vi "TDMS write test.vi"   [LabVIEW 2013]
types:
  T1 = enum16{"open", "open or create", "create or replace", "create", "open (read-only)"}
  T2 = typedef "electrical.ctl" = cluster{"date/time string":string, "Electrical Data Labels":string[], "Electrical Data":string[], "Waveform Graph":waveform(dbl)[]}
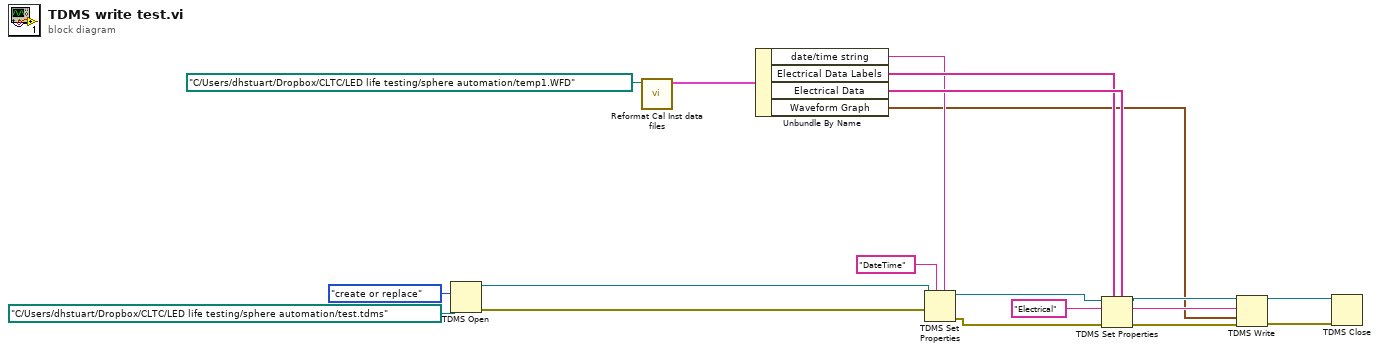
[diagram p0: block diagram]
diagram:
  n1 = TDMS Open(10:T1."create or replace" ("operation (0:open)"), 11:path "C:/Users/dhstuart/Dropbox/CLTC/LED life testing/sphere automation/test.tdms" ("file path")) -> (0:w17:errorcluster, 3:w18:refnum<k34>)  [unwired: 5 in]
  n2 = call "Reformat Cal Inst data files.vi"("file path (dialog if empty)"=path "C:/Users/dhstuart/Dropbox/CLTC/LED life testing/sphere automation/temp1.WFD") -> ("Electrical Data"=w15:T2)  [unwired: 10 in]
  n3 = Unbundle By Name(w15) -> ("date/time string"=w10:string, "Electrical Data Labels"=w12:string[], "Electrical Data"=w13:string[], "Waveform Graph"=w1:waveform(dbl)[])
  n4 = TDMS Set Properties(5:w10, 7:"DateTime" ("property names"), 8:w17, 11:w18) -> (0:w3:errorcluster, 3:w11:refnum<k34>)  [unwired: 2 in, 2 out]
  n5 = TDMS Set Properties(5:w13, 7:w12, 8:w3, 10:"Electrical" ("group name"), 11:w11) -> (0:w4:errorcluster, 2:w7:string, 3:w8:refnum<k34>)  [unwired: 1 in, 1 out]
  n6 = TDMS Write(0:w8, 5:w7, 9:w1, 11:w4) -> (4:w6:refnum<k34>, 15:w5:errorcluster)  [unwired: 2 in, 2 out]
  n7 = TDMS Close(8:w5, 11:w6) -> ()  [unwired: 2 out]
